vi "Temperature_Limit.vi"(3 "High Limit":dbl=80.0 format="%.2f", 4 "delta t (ms)":u32=400 min=50 max=2000 step=50, 5 "Points to Acquire":i32=75 min=20 max=500) -> ()   [LabVIEW 2016]
doc: "This VI simulates the acquisition of temperature, graphs the temperature, and notifies the user if the temperature is over the limit."
panel:
  out "Over Limit":bool
  in  "Abort":bool
  out "Temperature":cluster{"Temperature":dbl, "High Limit":dbl}(graph)
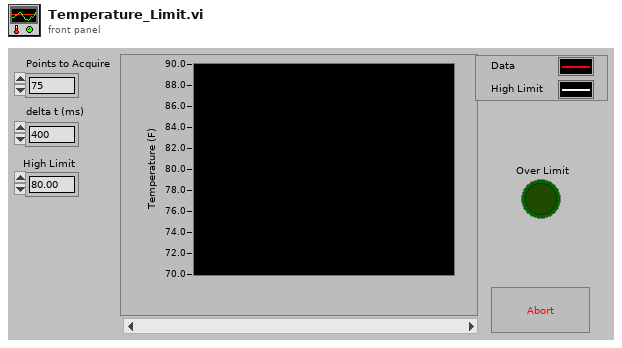
[diagram p1: front panel]
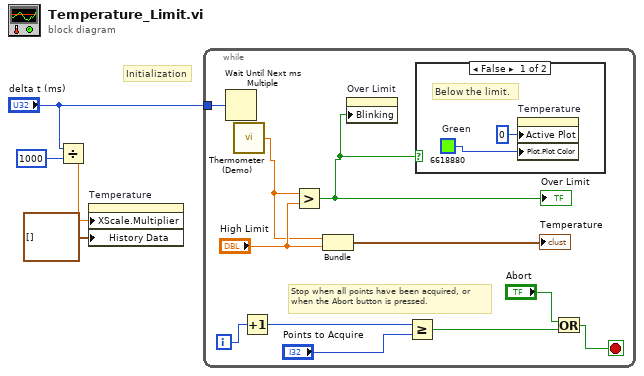
[diagram p0: block diagram]
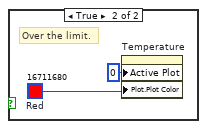
[diagram p2: hidden frame]
diagram:
  # "Initialization"
  n1 = Divide(x="delta t (ms)", y=u32 1000) -> (x/y=w3:dbl)
  n2 = property on="Temperature" class="WFChart (strict)"("XScale.Multiplier"=w3, "History Data"=cluster{"Temperature":dbl, "High Limit":dbl}[] []) -> ()  [unwired: 2 in, 2 out]
  n3 = while {
    tunnel: "delta t (ms)" -> [w7]
    i -> [w14]
    stop <- w8 stop-if-true
    # "Stop when all points have been acquired, or when the Abort button is pressed."
    n4 = Wait Until Next ms Multiple(millisecond multiple=w7) -> ()  [unwired: 1 out]
    n5 = call "Thermometer (Demo).vi"() -> ("Temperature"=w5:dbl)  [unwired: 1 in]
    n6 = Increment(x=w14) -> (x+1=w12:i32)
    n7 = Greater?(x=w5, y="High Limit") -> (0:w6:bool)
    "Over Limit" <- w6
    n8 = Bundle("Temperature"=w5, "High Limit"="High Limit") -> (→"Temperature":cluster{"Temperature":dbl, "High Limit":dbl})  [unwired: 1 in]
    n9 = property on="Over Limit" class="Bool (strict)"("Blinking"=w6) -> ()  [unwired: 2 in, 2 out]
    n10 = Greater Or Equal?(x=w12, y="Points to Acquire") -> (x >= y?=w10:bool)
    n11 = case shown="False" w6 {
      frame False {
        w17 = u32 6618880  # Green
        # "Below the limit."
        n12 = property on="Temperature" class="WFChart (strict)"("Active Plot"=u32 0, "Plot.Plot Color"=w17) -> ()  [unwired: 2 in, 2 out]
      }
      frame True {
        w18 = u32 16711680  # Red
        # "Over the limit."
        n13 = property on="Temperature" class="WFChart (strict)"("Active Plot"=u32 0, "Plot.Plot Color"=w18) -> ()  [unwired: 2 in, 2 out]
      }
    }
    n14 = Or(x="Abort", y=w10) -> (x .or. y?=w8:bool)
  }
